vi "set_config_cluster.vi"(8 "error in (no error)":errorcluster, 10 "config cluster variant":variant, 11 "StimulatorAK101022TCP in":refnum<class "StimulatorAK101022TCP.lvclass">) -> (0 "error out":errorcluster, 3 "StimulatorAK101022TCP out":refnum<class "StimulatorAK101022TCP.lvclass">)   [LabVIEW 2010, in "StimulatorAK101022TCP.lvclass"]
uses:
  StimulatorAK101022TCP.lvclass
  StimulatorAK101022TCP.lvclass/StimulatorAK101022TCP.ctl
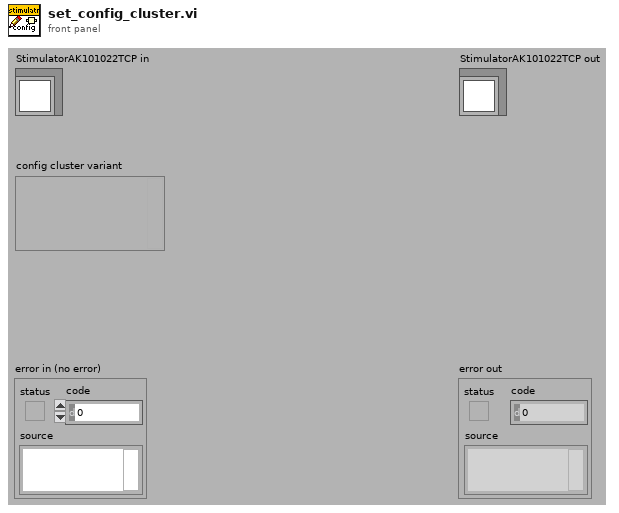
[diagram p1: front panel]
types:
  T1 = typedef "StimulatorAK101022TCP.lvclass/config_data_cluster.ctl" = cluster{"address":string, "port":u16, "stringGenerator":T2}
  T2 = typedef "plugin_specification.ctl" = cluster{"class path":string, "configuration":string, "label":string, "settings name":string}
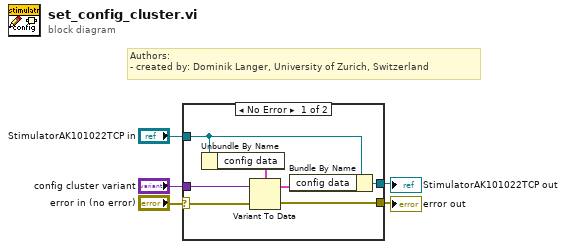
[diagram p0: block diagram]
diagram:
  # "Authors: \n- created by: Dominik Langer, University of Zurich, Switzerland"
  n1 = case shown="No Error" "error in (no error)" {
    selector: "error in (no error)" -> [w6 w13]
    tunnel: [w12 w13] -> w5
    tunnel: "config cluster variant" -> [w10 _]
    tunnel: "StimulatorAK101022TCP in" -> [w9 w14]
    tunnel: [w7 w14] -> w2
    frame No Error {
      n2 = Unbundle By Name(w9) -> ("config data"=w11:T1)
      n3 = Variant To Data(error in=w6, Variant=w10, type=w11) -> (error out=w12:errorcluster, data=w8:T1)
      n4 = Bundle By Name(cluster=w9, "config data"=w8) -> (w7:refnum<class "StimulatorAK101022TCP.lvclass">)
    }
    frame Error {
    }
  }
  "error out" <- w5
  "StimulatorAK101022TCP out" <- w2
